vi "Direction_Create.vi"(1 "dx":dbl=nan format="%.2f", 2 "dy":dbl=nan format="%.2f", 3 "p1":T1={"x"=nan, "y"=nan} {"y" format="%.2f"; "x" format="%.2f"}, 4 "p2":T1={"x"=nan, "y"=nan} {"y" format="%.2f"; "x" format="%.2f"}, 5 "error in (no error)":errorcluster) -> (14 "reference out":refnum<class "Direction.lvclass">, 19 "error out":errorcluster)   [LabVIEW 2016, in "Direction.lvclass"]
doc: "Creates and initializes a new Direction object.\n\nThis object should be destroyed using a Direction destructor VI.\n\n[GOOP 2.1]"
uses:
  <resource>/Framework/Providers/Open_GDS/UML/Direction_class/Direction.lvclass
  <resource>/Framework/Providers/Open_GDS/UML/General/Point/Point Point2D.ctl
  <resource>/Framework/Providers/Open_GDS/UML/Direction_class/Direction.lvclass/Direction.ctl
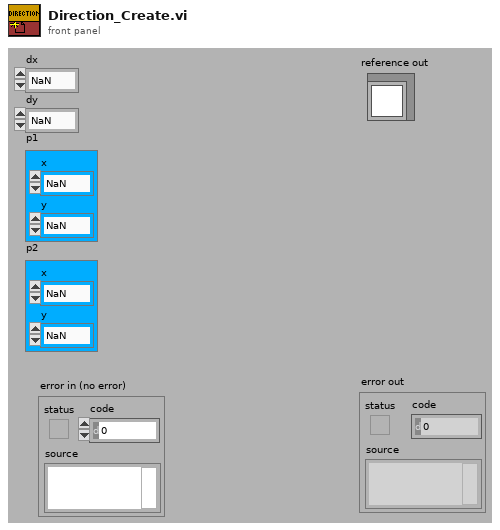
[diagram p1: front panel]
types:
  T1 = typedef "Point Point2D.ctl" = cluster{"x":dbl, "y":dbl}
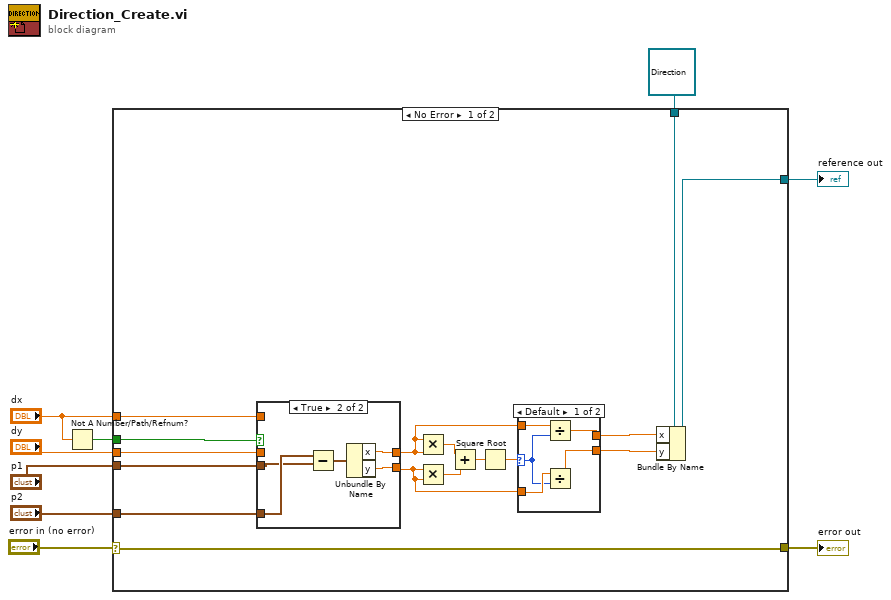
[diagram p0: block diagram]
diagram:
  n1 = Not A Number/Path/Refnum?(number/path/refnum="dx") -> (NaN/Path/Refnum?=w6:bool)
  n2 = case shown="No Error" "error in (no error)" {
    selector: "error in (no error)" -> [w11 w41]
    tunnel: [w12 w40] -> w9
    tunnel: [w11 w41] -> w8
    tunnel: w6 -> [w25 _]
    tunnel: "p1" -> [w24 _]
    tunnel: "p2" -> [w23 _]
    tunnel: "dx" -> [w22 _]
    tunnel: "dy" -> [w21 _]
    tunnel: refnum<class "Direction.lvclass"> refnum ("reference out") -> [w10 w40]
    frame No Error {
      n3 = case shown="True" w25 {
        tunnel: w24 -> [_ w38]
        tunnel: w23 -> [_ w39]
        tunnel: [w34 w36] -> w15
        tunnel: [w33 w35] -> w14
        tunnel: w22 -> [w34 _]
        tunnel: w21 -> [w33 _]
        frame False {
        }
        frame True {
          n4 = Subtract(x=w39, y=w38) -> (x-y=w37:T1)
          n5 = Unbundle By Name(w37) -> ("x"=w36:dbl, "y"=w35:dbl)
        }
      }
      n6 = Multiply(x=w15, y=w15) -> (x*y=w20:dbl)
      n7 = Multiply(x=w14, y=w14) -> (x*y=w19:dbl)
      n8 = Add(x=w20, y=w19) -> (x+y=w18:dbl)
      n9 = Square Root(x=w18) -> (sqrt(x)=w17:dbl)
      n10 = case shown="Default" w17 {
        selector: w17 -> [w27 _]
        tunnel: [w29 w32] -> w16
        tunnel: w15 -> [w30 w32]
        tunnel: w14 -> [w28 w31]
        tunnel: [w26 w31] -> w13
        frame Default {
          n11 = Divide(x=w30, y=w27) -> (x/y=w29:dbl)
          n12 = Divide(x=w28, y=w27) -> (x/y=w26:dbl)
        }
        frame 0 {
        }
      }
      n13 = Bundle By Name(cluster=w10, "x"=w16, "y"=w13) -> (w12:refnum<class "Direction.lvclass">)
    }
    frame Error {
    }
  }
  "error out" <- w8
  "reference out" <- w9
